vi "畫ROI.vi"(8 "error in (no error)":errorcluster, 10 "ROI In":T2, 11 "Image In":T1) -> (0 "error out":errorcluster, 3 "Image Out":T1)   [LabVIEW 2015]
uses:
  <vilib>/vision/Image Controls.llb/IMAQ Image.ctl
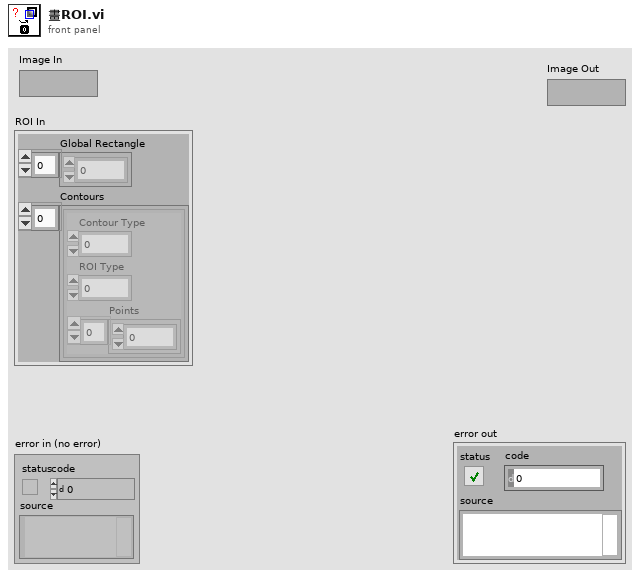
[diagram p1: front panel]
types:
  T1 = typedef "IMAQ Image.ctl" = refnum<image>
  T2 = cluster{"Global Rectangle":i32[], "Contours":cluster{"Contour Type":u32, "ROI Type":u32, "Points":i32[]}[]}
  T3 = typedef "ROI Descriptor" = cluster{"Global Rectangle":i32[], "Contours":cluster{"ID":enum32{"External", "Internal"}, "Type":u32, "Coordinates":i32[]}[]}
  T4 = cluster{"Contour Type":u32, "ROI Type":u32, "Points":i32[]}[]
  T5 = cluster{"Contour Type":u32, "ROI Type":u32, "Points":i32[]}
  T6 = cluster{"Left":i32, "Top":i32, "Right":i32, "Bottom":i32}
  T7 = typedef "IMAQ Point" = cluster{"X":sgl, "Y":sgl}
  T8 = typedef "IMAQ Line" = cluster{"Start X":i32, "Start Y":i32, "End X":i32, "End Y":i32}
  T9 = typedef "IMAQ Rectangle" = cluster{"Left":i32, "Top":i32, "Right":i32, "Bottom":i32, "Rotation":dbl}
  T10 = cluster{"Points[0]":i32, "Points[1]":i32, "Points[2]":i32, "Points[3]":i32, "Points[4]":i32}
  T11 = typedef "IMAQ Circle" = cluster{"Center X":i32, "Center Y":i32, "Inner Radius":i32, "Outer Radius":i32, "Start Angle":dbl, "End Angle":dbl}
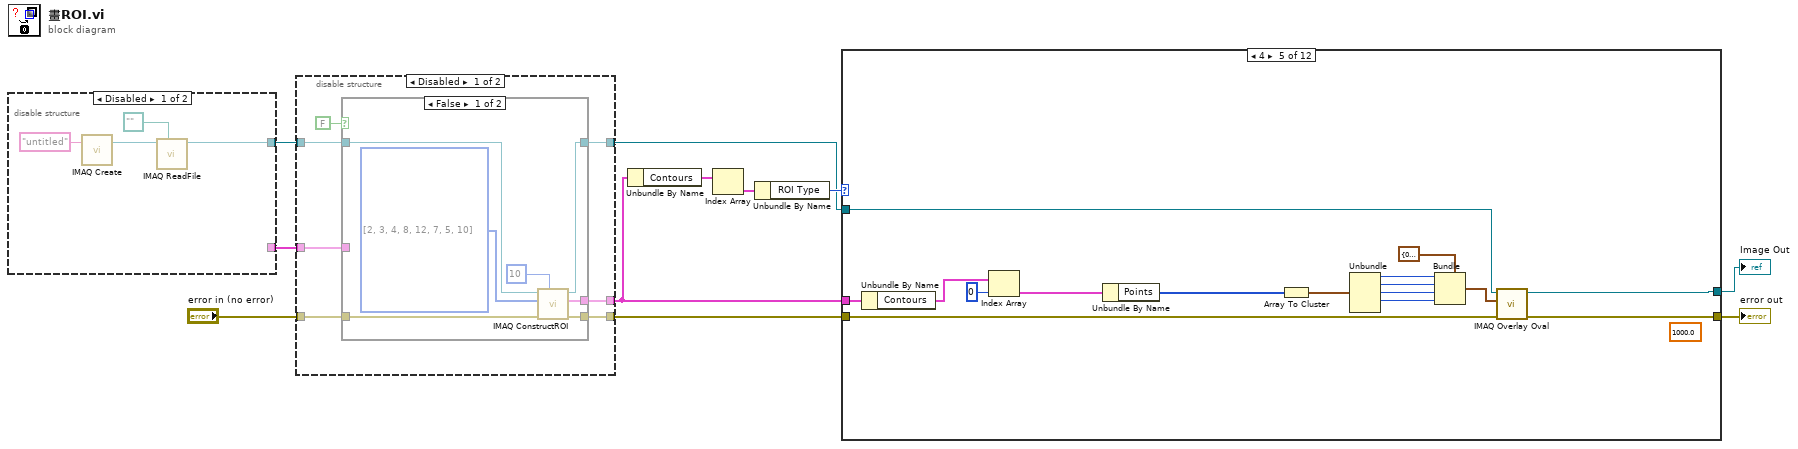
[diagram p0: block diagram]
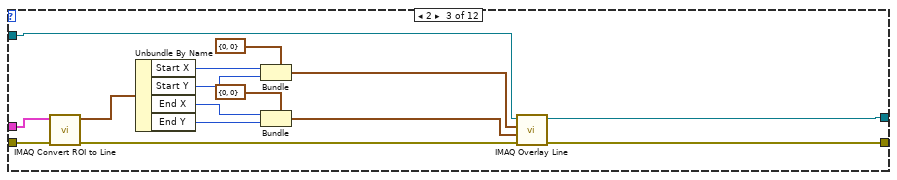
[diagram p6: hidden frame]
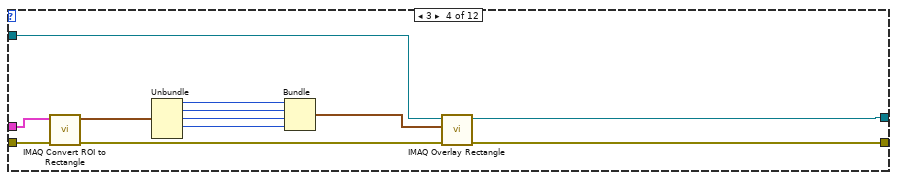
[diagram p7: hidden frame]
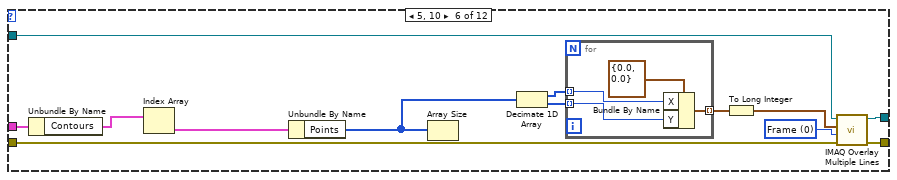
[diagram p8: hidden frame]
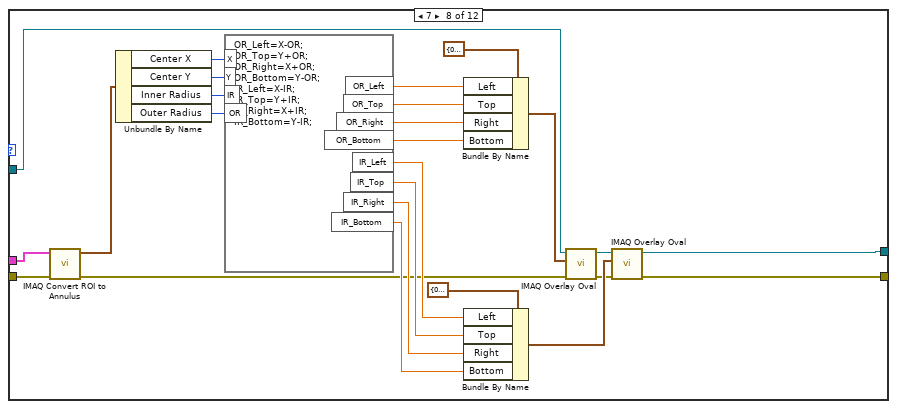
[diagram p10: hidden frame]
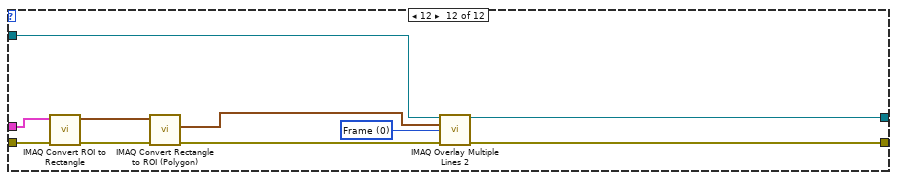
[diagram p14: hidden frame]
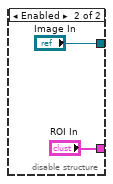
[diagram p15: hidden frame]
diagram:
  n1 = disable-structure shown="Disabled" {
    disable-tunnel: [w12 "Image In"] -> w7
    disable-tunnel: [_ "ROI In"] -> w3
    frame Disabled {
      n2 = call "IMAQ Create"("Image Name"="untitled") -> ("New Image"=w14:T1)  [unwired: 4 in, 1 out]
      n3 = call "IMAQ ReadFile"("File Path"=path "" ("Path"), "Image"=w14) -> ("Image Out"=w12:T1)  [unwired: 5 in, 4 out]
    }
    frame Enabled {
    }
  }
  n4 = disable-structure shown="Disabled" {
    disable-tunnel: w7 -> [w24 w37]
    disable-tunnel: [w23 w37] -> w6
    disable-tunnel: [w22 w36] -> w2
    disable-tunnel: "error in (no error)" -> [w21 w35]
    disable-tunnel: [w20 w35] -> w4
    disable-tunnel: w3 -> [w19 w36]
    frame Disabled {
      n5 = case shown="False" FALSE {
        tunnel: [w29 w34] -> w22
        tunnel: w19 -> [_ w34]
        tunnel: w24 -> [w28 w33]
        tunnel: [w27 w33] -> w23
        tunnel: w21 -> [w26 w32]
        tunnel: [w25 w32] -> w20
        frame False {
          w31 = u32[] [2, 3, 4, 8, 12, 7, 5, 10] items=["No Selection", "Point", "Line", "Rectangle", "Oval", "Polygon", "Freehand Region", "Annulus", "Zoom", "Pan", "Broken Line", "Freehand Line", "Rotated Rectangle"] ("Tools")
          n6 = call "IMAQ ConstructROI"("Window Number (-1...15)"=10, "error in (no error)"=w26, "Tools"=w31, "Image"=w28) -> ("error out"=w25:errorcluster, "ROI Descriptor Out"=w29:T3, "Image Out (duplicate)"=w27:T1)  [unwired: 4 in, 1 out]
        }
        frame True {
        }
      }
    }
    frame Enabled {
    }
  }
  n7 = Unbundle By Name(w2) -> ("Contours"=w11:T4)
  n8 = Index Array(array=w11) -> (element=w10:T5)  [unwired: 1 in]
  n9 = Unbundle By Name(w10) -> ("ROI Type"=w9:u32)
  n10 = case shown="4" w9 {
    tunnel: w6 -> [w39 w40 w55 w67 w83 w85 w101 w110 w127 w128 w129 w135]
    tunnel: [w39 w40 w54 w66 w82 w84 w101 w116 w127 w128 w129 w134] -> w1
    tunnel: w2 -> [_ _ w49 w59 w80 w96 _ w118 _ _ _ w139]
    tunnel: w4 -> [w38 _ w41 w58 w77 w88 _ w108 _ _ _ w133]
    tunnel: [w38 _ w43 w56 w76 w87 _ w105 _ _ _ w130] -> w8
    frame 0, Default {
    }
    frame 1 {
    }
    frame 2 {
      n11 = call "IMAQ Convert ROI to Line"("error in (no error)"=w41, "ROI Descriptor"=w49) -> ("error out"=w42:errorcluster, "Line"=w48:T8)  [unwired: 7 in]
      n12 = Unbundle By Name(w48) -> ("Start X"=w46:i32, "Start Y"=w47:i32, "End X"=w45:i32, "End Y"=w44:i32)
      n13 = Bundle(cluster=cluster{"X":i32, "Y":i32} {"X"=0, "Y"=0} ("Start Point"), "X"=w46, "Y"=w47) -> (w52:cluster{"X":i32, "Y":i32})
      n14 = Bundle(cluster=cluster{"X":i32, "Y":i32} {"X"=0, "Y"=0} ("Start Point"), "X"=w45, "Y"=w44) -> (w53:cluster{"X":i32, "Y":i32})
      n15 = call "IMAQ Overlay Line"("error in (no error)"=w42, "End Point"=w53, "Start Point"=w52, "Image"=w55) -> ("error out"=w43:errorcluster, "Image Out"=w54:T1)  [unwired: 6 in]
    }
    frame 3 {
      n16 = call "IMAQ Convert ROI to Rectangle"("error in (no error)"=w58, "ROI Descriptor"=w59) -> ("error out"=w57:errorcluster, "Rectangle"=w61:T9)  [unwired: 7 in]
      n17 = Unbundle(w61) -> ("Left"=w62:i32, "Top"=w63:i32, "Right"=w64:i32, "Bottom"=w65:i32)  [unwired: 1 out]
      n18 = Bundle("Left"=w62, "Top"=w63, "Right"=w64, "Bottom"=w65) -> (w60:T6)  [unwired: 1 in]
      n19 = call "IMAQ Overlay Rectangle"("error in (no error)"=w57, "Rectangle"=w60, "Image"=w67) -> ("error out"=w56:errorcluster, "Image Out"=w66:T1)  [unwired: 7 in]
    }
    frame 4 {
      (unwired) 1000.0 ("y")
      n20 = Unbundle By Name(w80) -> ("Contours"=w78:T4)
      n21 = Index Array(array=w78, index=0 ("Index")) -> (element=w69:T5)
      n22 = Unbundle By Name(w69) -> ("Points"=w68:i32[])
      n23 = Array To Cluster(array=w68) -> (cluster=w75:T10)
      n24 = Unbundle(w75) -> ("Points[0]"=w74:i32, "Points[1]"=w73:i32, "Points[2]"=w72:i32, "Points[3]"=w71:i32)  [unwired: 1 out]
      n25 = Bundle(cluster=T6 {"Left"=0, "Top"=0, "Right"=0, "Bottom"=0} ("Bounding Rectangle"), "Left"=w74, "Top"=w73, "Right"=w72, "Bottom"=w71) -> (w81:T6)
      n26 = call "IMAQ Overlay Oval"("error in (no error)"=w77, "Bounding Rectangle"=w81, "Image"=w83) -> ("error out"=w76:errorcluster, "Image Out"=w82:T1)  [unwired: 7 in]
    }
    frame 5, 10 {
      w89 = u32 0 items=["Frame", "Fill"] ("Drawing Mode (Frame)")
      n27 = Unbundle By Name(w96) -> ("Contours"=w95:T4)
      n28 = Index Array(array=w95) -> (element=w94:T5)  [unwired: 1 in]
      n29 = Unbundle By Name(w94) -> ("Points"=w93:i32[])
      n30 = Array Size(array=w93) -> ()  [unwired: 1 out]
      n31 = Decimate 1D Array(w93) -> (w92:i32[], w91:i32[])
      n32 = for {
        tunnel: w92 -> [w99] mode=indexing
        tunnel: w91 -> [w98] mode=indexing
        tunnel: [w97] -> w86 mode=indexing
        n33 = Bundle By Name(cluster=T7 {"X"=0.0, "Y"=0.0} ("Point"), "X"=w99, "Y"=w98) -> (w97:T7)
      }
      n34 = To Long Integer(number=w86) -> (32bit integer=w90:cluster{"X":i32, "Y":i32}[])
      n35 = call "IMAQ Overlay Multiple Lines"("error in (no error)"=w88, "Drawing Mode (Frame)"=w89, "Line End Points"=w90, "Image"=w85) -> ("error out"=w87:errorcluster, "Image Out"=w84:T1)  [unwired: 2 in, 4 out]
    }
    frame 6 {
    }
    frame 7 {
      n36 = call "IMAQ Convert ROI to Annulus"("error in (no error)"=w108, "ROI Descriptor"=w118) -> ("error out"=w107:errorcluster, "Annulus"=w126:T11)  [unwired: 7 in]
      n37 = Unbundle By Name(w126) -> ("Center X"=w125:i32, "Center Y"=w124:i32, "Inner Radius"=w123:i32, "Outer Radius"=w122:i32)
      n38 = formula code="OR_Left=X-OR;\nOR_Top=Y+OR;\nOR_Right=X+OR;\nOR_Bottom=Y-OR;\nIR_Left=X-IR;\nIR_Top=Y+IR;\nIR_Right=X+IR;\nIR_Bottom=Y-IR;"("X"=w125, "Y"=w124, "IR"=w123, "OR"=w122) -> ("OR_Left"=w121:dbl, "OR_Top"=w103:dbl, "OR_Right"=w102:dbl, "OR_Bottom"=w120:dbl, "IR_Left"=w114:dbl, "IR_Top"=w113:dbl, "IR_Right"=w112:dbl, "IR_Bottom"=w111:dbl)
      n39 = Bundle By Name(cluster=T6 {"Left"=0, "Top"=0, "Right"=0, "Bottom"=0} ("Bounding Rectangle"), "Left"=w121, "Top"=w103, "Right"=w102, "Bottom"=w120) -> (w119:T6)
      n40 = Bundle By Name(cluster=T6 {"Left"=0, "Top"=0, "Right"=0, "Bottom"=0} ("Bounding Rectangle"), "Left"=w114, "Top"=w113, "Right"=w112, "Bottom"=w111) -> (w117:T6)
      n41 = call "IMAQ Overlay Oval"("error in (no error)"=w107, "Bounding Rectangle"=w119, "Image"=w110) -> ("error out"=w106:errorcluster, "Image Out"=w109:T1)  [unwired: 7 in]
      n42 = call "IMAQ Overlay Oval"("error in (no error)"=w106, "Bounding Rectangle"=w117, "Image"=w109) -> ("error out"=w105:errorcluster, "Image Out"=w116:T1)  [unwired: 7 in]
    }
    frame 8 {
    }
    frame 9 {
    }
    frame 11 {
    }
    frame 12 {
      w136 = u32 0 items=["Frame", "Fill"] ("Drawing Mode (Frame)")
      n43 = call "IMAQ Convert ROI to Rectangle"("error in (no error)"=w133, "ROI Descriptor"=w139) -> ("error out"=w132:errorcluster, "Rectangle"=w138:T9)  [unwired: 7 in]
      n44 = call "IMAQ Convert Rectangle to ROI (Polygon)"("error in (no error)"=w132, "Rectangle"=w138) -> ("error out"=w131:errorcluster, "Rectangle Points"=w137:T7[])  [unwired: 6 in, 1 out]
      n45 = call "IMAQ Overlay Multiple Lines 2"("Image"=w135, "Line End Points"=w137, "Drawing Mode (Frame)"=w136, "error in (no error)"=w131) -> ("Image Out"=w134:T1, "error out"=w130:errorcluster)  [unwired: 10 in]
    }
  }
  "error out" <- w8
  "Image Out" <- w1
